vi "SW_get_IO_ports_representation_2.vi"(1 "Sync parameters cluster input":T2={"IO general config."=12, "IO 1 configuration"=1, "IO 2 configuration"=1, "IO 3 configuration"=0, "IO 4 configuration"=0, "Activate ext. RS-232"=0, "IO inversion config."=0, "Sync capability"=0}) -> (0 "IO status indicator":T1)   [LabVIEW 2018, in "Tracker.lvlib"]
uses:
  Tracker.lvlib
  Controls/CTL_IO_params_cluster.ctl
  Controls/CTL_IO_status_indicator.ctl
  <vilib>/Utility/miscctls.llb/LVPointTypeDef.ctl
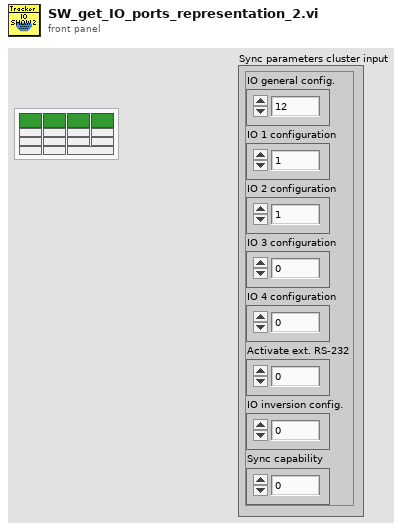
[diagram p1: front panel]
types:
  T1 = typedef "Tracker.lvlib/CTL_IO_status_indicator.ctl" = cluster{"IO1":bool, "IO2":bool, "IO3":bool, "IO4":bool, "St1":bool, "St2":bool, "St3":bool, "St4":bool, "Z1":bool, "Z2":bool, "Z3":bool, "Z4":bool, "Syn1":bool, "Syn2":bool, "RS-232 ext. activated":bool}
  T2 = typedef "Tracker.lvlib/CTL_IO_params_cluster.ctl" = cluster{"IO general config.":u16, "IO 1 configuration":u16, "IO 2 configuration":u16, "IO 3 configuration":u16, "IO 4 configuration":u16, "Activate ext. RS-232":u16, "IO inversion config.":u16, "Sync capability":u8}
  T3 = typedef "LVPointTypeDef.ctl" = cluster{"Horizontal":i16, "Vertical":i16}
  T4 = cluster{"IO1":bool, "IO2":bool, "IO3":bool, "IO4":bool, "Z1":bool, "Z2":bool, "Z3":bool, "Z4":bool, "St1":bool, "St2":bool, "St3":bool, "St4":bool, "Syn1":bool, "Syn2":bool, "RS-232 ext. activated":bool}
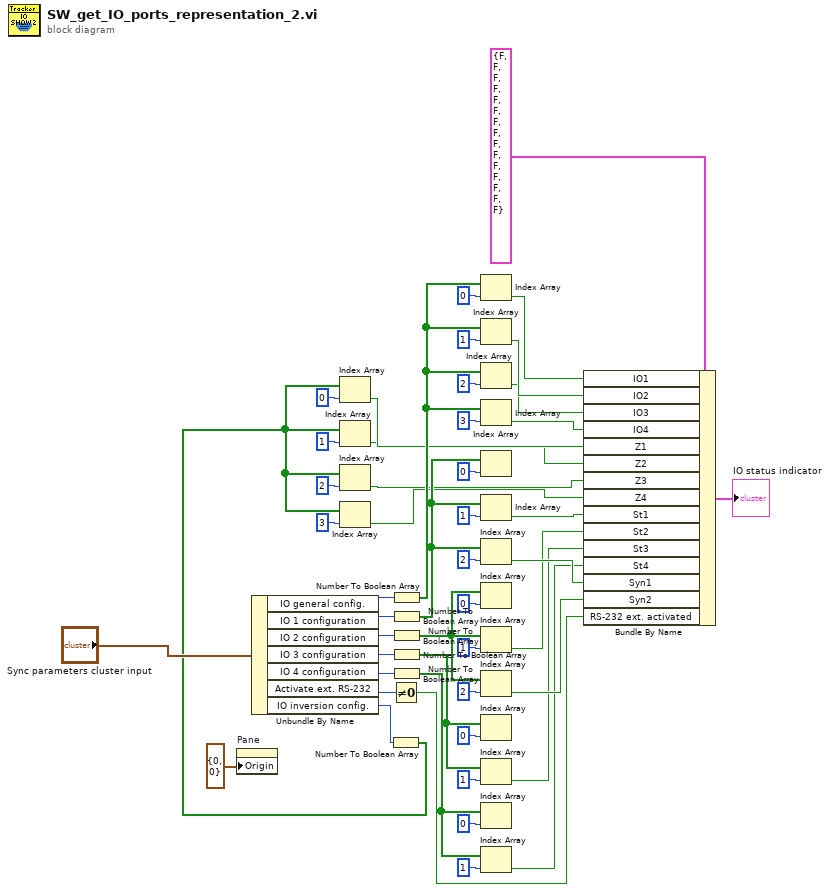
[diagram p0: block diagram]
diagram:
  n1 = property on="Pane" class="Pane"("Origin"=T3 {"Horizontal"=0, "Vertical"=0}) -> ()  [unwired: 2 in, 2 out]
  n2 = Unbundle By Name("Sync parameters cluster input") -> ("IO general config."=w37:u16, "IO 1 configuration"=w31:u16, "IO 2 configuration"=w22:u16, "IO 3 configuration"=w17:u16, "IO 4 configuration"=w16:u16, "Activate ext. RS-232"=w15:u16, "IO inversion config."=w10:u16)
  n3 = Not Equal To 0?(x=w15) -> (x != 0?=w38:bool)
  n4 = Number To Boolean Array(number=w10) -> (Boolean array=w5:bool[])
  n5 = Index Array(array=w5, index=0) -> (element=w4:bool)
  n6 = Index Array(array=w5, index=1) -> (element=w3:bool)
  n7 = Index Array(array=w5, index=2) -> (element=w2:bool)
  n8 = Index Array(array=w5, index=3) -> (element=w1:bool)
  n9 = Number To Boolean Array(number=w37) -> (Boolean array=w36:bool[])
  n10 = Number To Boolean Array(number=w31) -> (Boolean array=w30:bool[])
  n11 = Number To Boolean Array(number=w22) -> (Boolean array=w23:bool[])
  n12 = Number To Boolean Array(number=w17) -> (Boolean array=w21:bool[])
  n13 = Number To Boolean Array(number=w16) -> (Boolean array=w18:bool[])
  n14 = Index Array(array=w36, index=0) -> (element=w49:bool)
  n15 = Index Array(array=w36, index=1) -> (element=w48:bool)
  n16 = Index Array(array=w36, index=2) -> (element=w47:bool)
  n17 = Index Array(array=w36, index=3) -> (element=w46:bool)
  n18 = Index Array(array=w30, index=0) -> ()  [unwired: 1 out]
  n19 = Index Array(array=w30, index=1) -> (element=w44:bool)
  n20 = Index Array(array=w30, index=2) -> (element=w43:bool)
  n21 = Index Array(array=w23, index=0) -> ()  [unwired: 1 out]
  n22 = Index Array(array=w23, index=1) -> (element=w42:bool)
  n23 = Index Array(array=w23, index=2) -> (element=w41:bool)
  n24 = Index Array(array=w21, index=0) -> ()  [unwired: 1 out]
  n25 = Index Array(array=w21, index=1) -> (element=w40:bool)
  n26 = Index Array(array=w18, index=0) -> ()  [unwired: 1 out]
  n27 = Index Array(array=w18, index=1) -> (element=w39:bool)
  n28 = Bundle By Name(cluster=T4 {"IO1"=FALSE, "IO2"=FALSE, "IO3"=FALSE, "IO4"=FALSE, "Z1"=FALSE, "Z2"=FALSE, "Z3"=FALSE, "Z4"=FALSE, "St1"=FALSE, "St2"=FALSE, "St3"=FALSE, "St4"=FALSE, "Syn1"=FALSE, "Syn2"=FALSE, "RS-232 ext. activated"=FALSE} ("IO status indicator 2"), "IO1"=w49, "IO2"=w48, "IO3"=w47, "IO4"=w46, "Z1"=w4, "Z2"=w3, "Z3"=w2, "Z4"=w1, "St1"=w44, "St2"=w42, "St3"=w40, "St4"=w39, "Syn1"=w43, "Syn2"=w41, "RS-232 ext. activated"=w38) -> (→"IO status indicator":T4)
